vi "pump_initial.vi"(8 "error in (no error)":errorcluster, 11 "Serial Port in":refnum<visa-resource-name>) -> (0 "error out":errorcluster, 3 "Serial Port out":refnum<visa-resource-name>)   [LabVIEW 2020]
uses:
  <vilib>/Instr/_visa.llb/VISA Configure Serial Port (Instr).vi
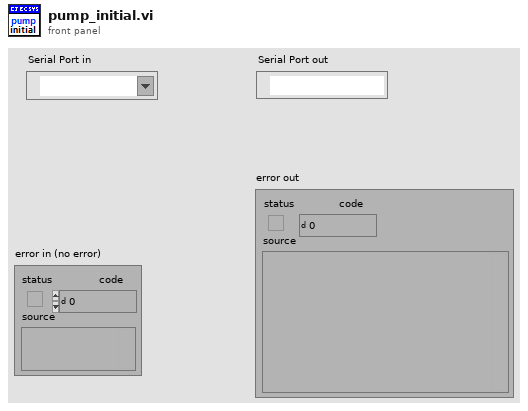
[diagram p1: front panel]
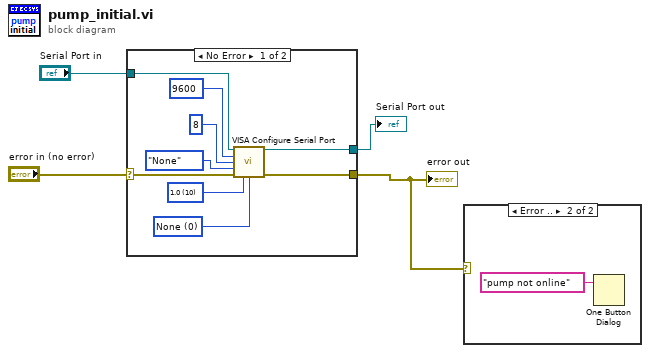
[diagram p0: block diagram]
diagram:
  n1 = case shown="No Error" "error in (no error)" {
    selector: "error in (no error)" -> [w8 w15]
    tunnel: "Serial Port in" -> [w13 w14]
    tunnel: [w7 w14] -> w3
    tunnel: [w6 w15] -> w1
    frame No Error {
      w9 = u16 10 items=["1.0"=10, "1.5"=15, "2.0"=20] ("stop bits (10: 1 bit)")
      w10 = u16 0 items=["None", "XON/XOFF", "RTS/CTS", "XON/XOFF & RTS/CTS", "DTR/DSR", "XON/XOFF & DTR/DSR"] ("flow control (0:none)")
      n2 = call-poly "VISA Configure Serial Port"("VISA resource name"=w13, "baud rate (9600)"=u32 9600, "data bits (8)"=u16 8, "parity (0:none)"=enum16{"None", "Odd", "Even", "Mark", "Space"}."None", "error in (no error)"=w8, "stop bits (10: 1 bit)"=w9, "flow control (0:none)"=w10) -> ("VISA resource name out"=w7:refnum<visa-resource-name>, "error out"=w6:errorcluster)  [unwired: 7 in]
    }
    frame Error {
      # "Error in: no initialization"
    }
  }
  "Serial Port out" <- w3
  "error out" <- w1
  n3 = case shown="Error .." w1 {
    frame No Error {
    }
    frame Error {
      n4 = One Button Dialog(message="pump not online") -> ()  [unwired: 1 in, 1 out]
    }
  }
